vi "SLSCTest Datatype Conversion.vi"() -> (3 "Passed?":bool)   [LabVIEW 2015, in "SLSC EDS Testing.lvlib"]
uses:
  SLSC EDS Testing.lvlib
  <vilib>/Utility/Data Type/Type Definitions/Data Type.ctl
  SLSC UI API/SLSC Tree Control.lvlib
  <vilib>/Utility/Data Type/NI_Data Type.lvlib
panel:
  out "Command":bool[](array[boolean])
  out "Numeric":i32
  out "U64 2":u64
  out "U64":u64
  out "I32":i32
  out "I8":i8
  out "I64":i64
  out "Reset Variant Check":bool[](array[boolean])
  out "Reset = Value?":bool[](array[boolean])
  out "Value Variant Check":bool[](array[boolean])
  out "String Comparison":bool[](array[boolean])
  out "Value (DBL)":dbl format="%#_16f"
  out "Type":T1
  in  "Ring":u16(ring)
  out "NewVal":variant
  out "Value 2 (DBL)":dbl format="%#_16f"
  out "Value":variant
  out "string data value":string
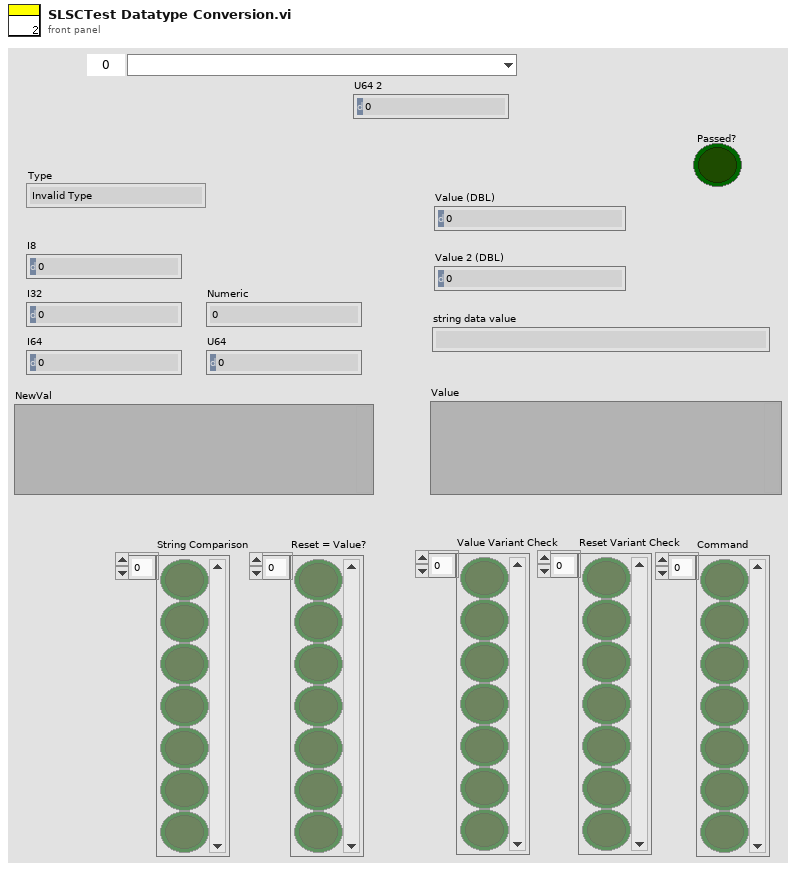
[diagram p1: front panel]
types:
  T1 = typedef "NI_Data Type.lvlib/Data Type.ctl" = enum8{"Invalid Type", "Void", "I8", "I16", "I32", "I64", "U8", "U16", "U32", "U64", "Single Float", "Double Float", "Extended Float", "Single Complex", "Double Complex", "Extended Complex", "Enum U8", "Enum U16", "Enum U32", "Enum U64", "Single Float With Unit", "Double Float With Unit", "Extended Float With Unit", "Single Complex with Unit", "Double Complex with Unit", "Extended Complex with Unit", "Boolean", "String", "Path", "Picture", "Tag", "Array", "Cluster", "Variant", "LV Variant", "Waveform", "Timestamp", "Digital Waveform", "Digital Data", "ExpressData", "Refnum", "External Data", "VI", "Poly VI", "LabVIEW Class Instance", "Fixed Point"}
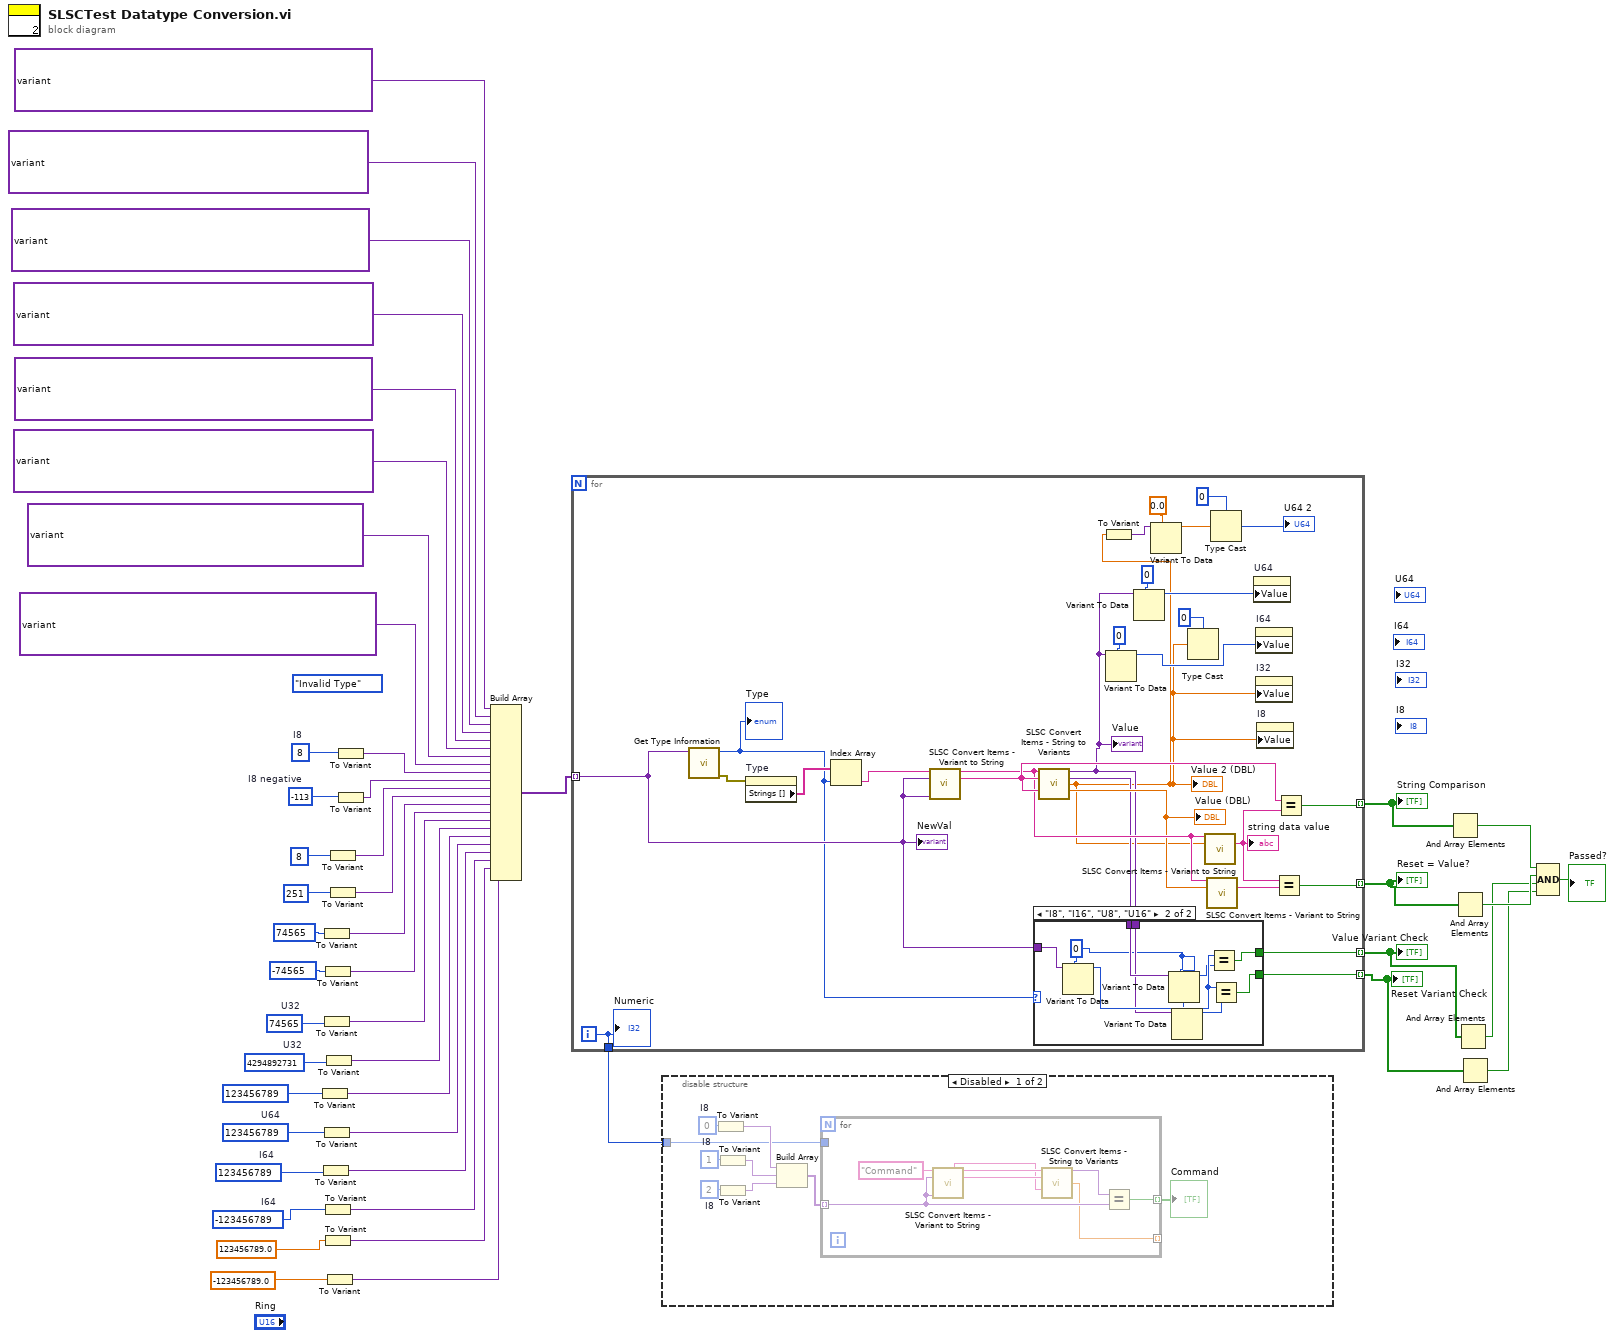
[diagram p0: block diagram]
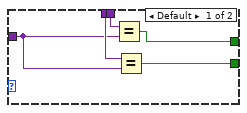
[diagram p3: hidden frame]
diagram:
  w30 = i64 -123456789  # I64
  w32 = u64 123456789  # U64
  w29 = i64 123456789  # I64
  w33 = u32 4294892731  # U32
  w34 = u32 74565  # U32
  (unwired) Data_Type."Invalid Type" ("Type")
  w46 = i8 -113  # I8 negative
  w47 = i8 8  # I8
  n1 = To Variant(anything=u64 123456789 ("U64")) -> (Variant=w26:variant)
  n2 = To Variant(anything=w29) -> (Variant=w24:variant)
  n3 = To Variant(anything=74565 ("I32")) -> (Variant=w37:variant)
  n4 = To Variant(anything=w34) -> (Variant=w28:variant)
  n5 = To Variant(anything=w32) -> (Variant=w25:variant)
  n6 = To Variant(anything=-74565 ("I32")) -> (Variant=w35:variant)
  n7 = To Variant(anything=w30) -> (Variant=w23:variant)
  n8 = To Variant(anything=123456789.0 ("DBL")) -> (Variant=w20:variant)
  n9 = To Variant(anything=w33) -> (Variant=w27:variant)
  n10 = To Variant(anything=-123456789.0 ("DBL")) -> (Variant=w19:variant)
  n11 = To Variant(anything=u8 8 ("U8")) -> (Variant=w41:variant)
  n12 = To Variant(anything=u8 251 ("U8")) -> (Variant=w39:variant)
  n13 = To Variant(anything=w47) -> (Variant=w45:variant)
  n14 = To Variant(anything=w46) -> (Variant=w44:variant)
  n15 = Build Array(variant(i32 -15) ("variant"), variant(u32 241) ("variant"), variant(i32 -3343) ("variant"), variant(u32 62193) ("variant"), variant(i32 -185339151) ("variant"), variant(u32 4109628145) ("variant"), variant(i64 -506664896818842895) ("variant"), variant(u64 17940079176890708721) ("variant"), w45, w44, w41, w39, w37, w35, w28, w27, w26, w25, w24, w23, w20, w19) -> (w43:variant[])
  n16 = for {
    tunnel: w43 -> [w63] mode=indexing
    tunnel: [w67] -> w10 mode=indexing
    tunnel: [w66] -> w9 mode=indexing
    tunnel: [w65] -> w8 mode=indexing
    tunnel: [w62] -> w7 mode=indexing
    tunnel: [w48] -> w1
    i -> [w48]
    n17 = call <vilib>:"Get Type Information.vi"("Variant"=w63) -> ("error out"=w75:errorcluster, "Type"=w56:T1)  [unwired: 6 in, 3 out]
    "Type" <- w56
    n18 = property on="Type" class="Enum (strict)"(error in=w75) -> ("Strings []"=w74:string[])  [unwired: 1 in, 2 out]
    n19 = Index Array(array=w74, index=w56) -> (element=w73:string)
    n20 = call "SLSC Convert Items - Variant to String.vi"("Datatype"=w73, "value"=w63, "reset value"=w63) -> ("Output data type"=w71:string, "string data value"=w72:string)  [unwired: 6 in, 5 out]
    n21 = call "SLSC Convert Items - String to Variants.vi"("Datatype"=w71, "Value"=w72, "Reset Value"=w72) -> ("Value"=w53:variant, "Reset Value"=w64:variant, "Value (DBL)"=w50:dbl, "Reset Value (DBL)"=w70:dbl)  [unwired: 9 in]
    "Value 2 (DBL)" <- w50
    "Value" <- w53
    "Value (DBL)" <- w70
    n22 = case shown="\"I8\", \"I16\", \"U8\", \"U16\"" w56 {
      tunnel: [w80 w85] -> w65
      tunnel: w64 -> [w79 w88]
      tunnel: w63 -> [w78 w89]
      tunnel: [w77 w83] -> w62
      tunnel: w53 -> [w76 w84]
      frame Default {
        n23 = Equal?(x=w76, y=w78) -> (x = y?=w80:bool)
        n24 = Equal?(x=w79, y=w78) -> (x = y?=w77:bool)
      }
      frame "I8", "I16", "U8", "U16" {
        w81 = i64 0
        n25 = Variant To Data(type=w81, Variant=w89) -> (data=w87:i64)  [unwired: 1 in, 1 out]
        n26 = Variant To Data(type=w81, Variant=w88) -> (data=w86:i64)  [unwired: 1 in, 1 out]
        n27 = Variant To Data(type=w81, Variant=w84) -> (data=w82:i64)  [unwired: 1 in, 1 out]
        n28 = Equal?(x=w87, y=w86) -> (x = y?=w85:bool)
        n29 = Equal?(x=w87, y=w82) -> (x = y?=w83:bool)
      }
    }
    n30 = To Variant(anything=w50) -> (Variant=w49:variant)
    n31 = Variant To Data(type=i64 0, Variant=w53) -> (data=w59:i64)  [unwired: 1 in, 1 out]
    n32 = Variant To Data(type=u64 0, Variant=w53) -> (data=w57:u64)  [unwired: 1 in, 1 out]
    n33 = Variant To Data(type=0.0, Variant=w49) -> (data=w54:dbl)  [unwired: 1 in, 1 out]
    n34 = Type Cast(type=i64 0 ("I64"), x=w50) -> ()  [unwired: 1 out]
    n35 = call "SLSC Convert Items - Variant to String.vi"("Datatype"=w71, "value"=w50) -> ("string data value"=w68:string)  [unwired: 7 in, 6 out]
    "string data value" <- w68
    n36 = call "SLSC Convert Items - Variant to String.vi"("Datatype"=w71, "value"=w70) -> ("string data value"=w69:string)  [unwired: 7 in, 6 out]
    n37 = Type Cast(type=i64 0, x=w54) -> (*(type *) &x=→"U64 2":i64)
    n38 = property on="U64" class="DigNum (strict)"("Value"=w57) -> ()  [unwired: 2 in, 2 out]
    n39 = property on="I64" class="DigNum (strict)"("Value"=w59) -> ()  [unwired: 2 in, 2 out]
    n40 = property on="I32" class="DigNum (strict)"("Value"=w50) -> ()  [unwired: 2 in, 2 out]
    n41 = property on="I8" class="DigNum (strict)"("Value"=w50) -> ()  [unwired: 2 in, 2 out]
    n42 = Equal?(x=w68, y=w69) -> (x = y?=w66:bool)
    n43 = Equal?(x=w72, y=w68) -> (x = y?=w67:bool)
    "NewVal" <- w63
    "Numeric" <- w48
  }
  "String Comparison" <- w10
  "Value Variant Check" <- w8
  "Reset = Value?" <- w9
  "Reset Variant Check" <- w7
  n44 = disable-structure shown="Disabled" {
    disable-tunnel: w1 -> [w90 _]
    frame Disabled {
      w94 = i8 2  # I8
      w96 = i8 1  # I8
      w98 = i8 0  # I8
      n45 = To Variant(anything=w98) -> (Variant=w97:variant)
      n46 = To Variant(anything=w96) -> (Variant=w95:variant)
      n47 = To Variant(anything=w94) -> (Variant=w93:variant)
      n48 = Build Array(w97, w95, w93) -> (w92:variant[])
      n49 = for {
        tunnel: w92 -> [w102] mode=indexing
        tunnel: [w101] -> w91 mode=indexing
        tunnel: [w100] -> _ mode=indexing
        tunnel: w90 -> [_]
        n50 = call "SLSC Convert Items - Variant to String.vi"("Datatype"="Command", "value"=w102, "reset value"=w102) -> ("string data reset value"=w99:string, "Output data type"=w106:string, "string data value"=w105:string)  [unwired: 6 in, 4 out]
        n51 = call "SLSC Convert Items - String to Variants.vi"("Datatype"=w106, "Value"=w105, "Reset Value"=w99) -> ("Value"=w103:variant, "Value (DBL)"=w100:dbl)  [unwired: 9 in, 2 out]
        n52 = Equal?(x=w103, y=w102) -> (x = y?=w101:bool)
      }
      "Command" <- w91
    }
    frame Enabled {
    }
  }
  n53 = And Array Elements(Boolean array=w10) -> (logical AND=w6:bool)
  n54 = And Array Elements(Boolean array=w9) -> (logical AND=w5:bool)
  n55 = And Array Elements(Boolean array=w8) -> (logical AND=w4:bool)
  n56 = And Array Elements(Boolean array=w7) -> (logical AND=w3:bool)
  n57 = Compound Arithmetic op=AND(w6, w5, w4, w3) -> (→"Passed?":bool)
